vi "save_infos_v4_svi.vi"(0 "Refnum VISA en entrée":refnum<visa-resource-name>, 1 "STAGE_SPEED":dbl, 2 "info Directory":path, 3 "USED_FILTERS":u8[](array[numeric]), 4 "NUM_POS":u32, 5 "NB_CHANELS":u32, 6 "NSCAN":u32, 7 "Noff_fluidix":u32, 8 "Camera infos":string, 9 "BETWEEN_SCAN":u32, 10 "ROMODE":u32, 11 "Non_fluidix":u32, 12 "BIN":u16, 13 "useLASER":bool, 14 "SOFT_VERSION":string, 15 "Nstart_fluidics":u32, 16 "EXPT":dbl, 17 "MIN SCAN DURATION":dbl, 18 "USED_LEDS":bool[][](array[boolean]), 19 "useFLUIDCS":bool, 20 "Noff_laser":u32, 21 "Non_laser":u32, 22 "Nstart_laser":u32, 23 "BETWEEN_PATTERN":u32, 24 "NPATTERN":u32, 25 "SHOOT_AT_SCAN":u32, 26 "SHOOT_DUR":dbl, 27 "is_singleshoot":bool) -> ()   [LabVIEW 2013]
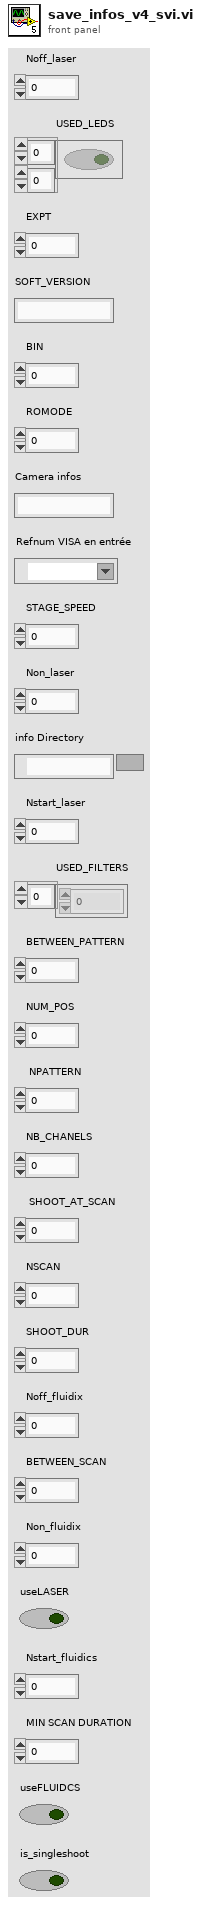
[diagram p1: front panel]
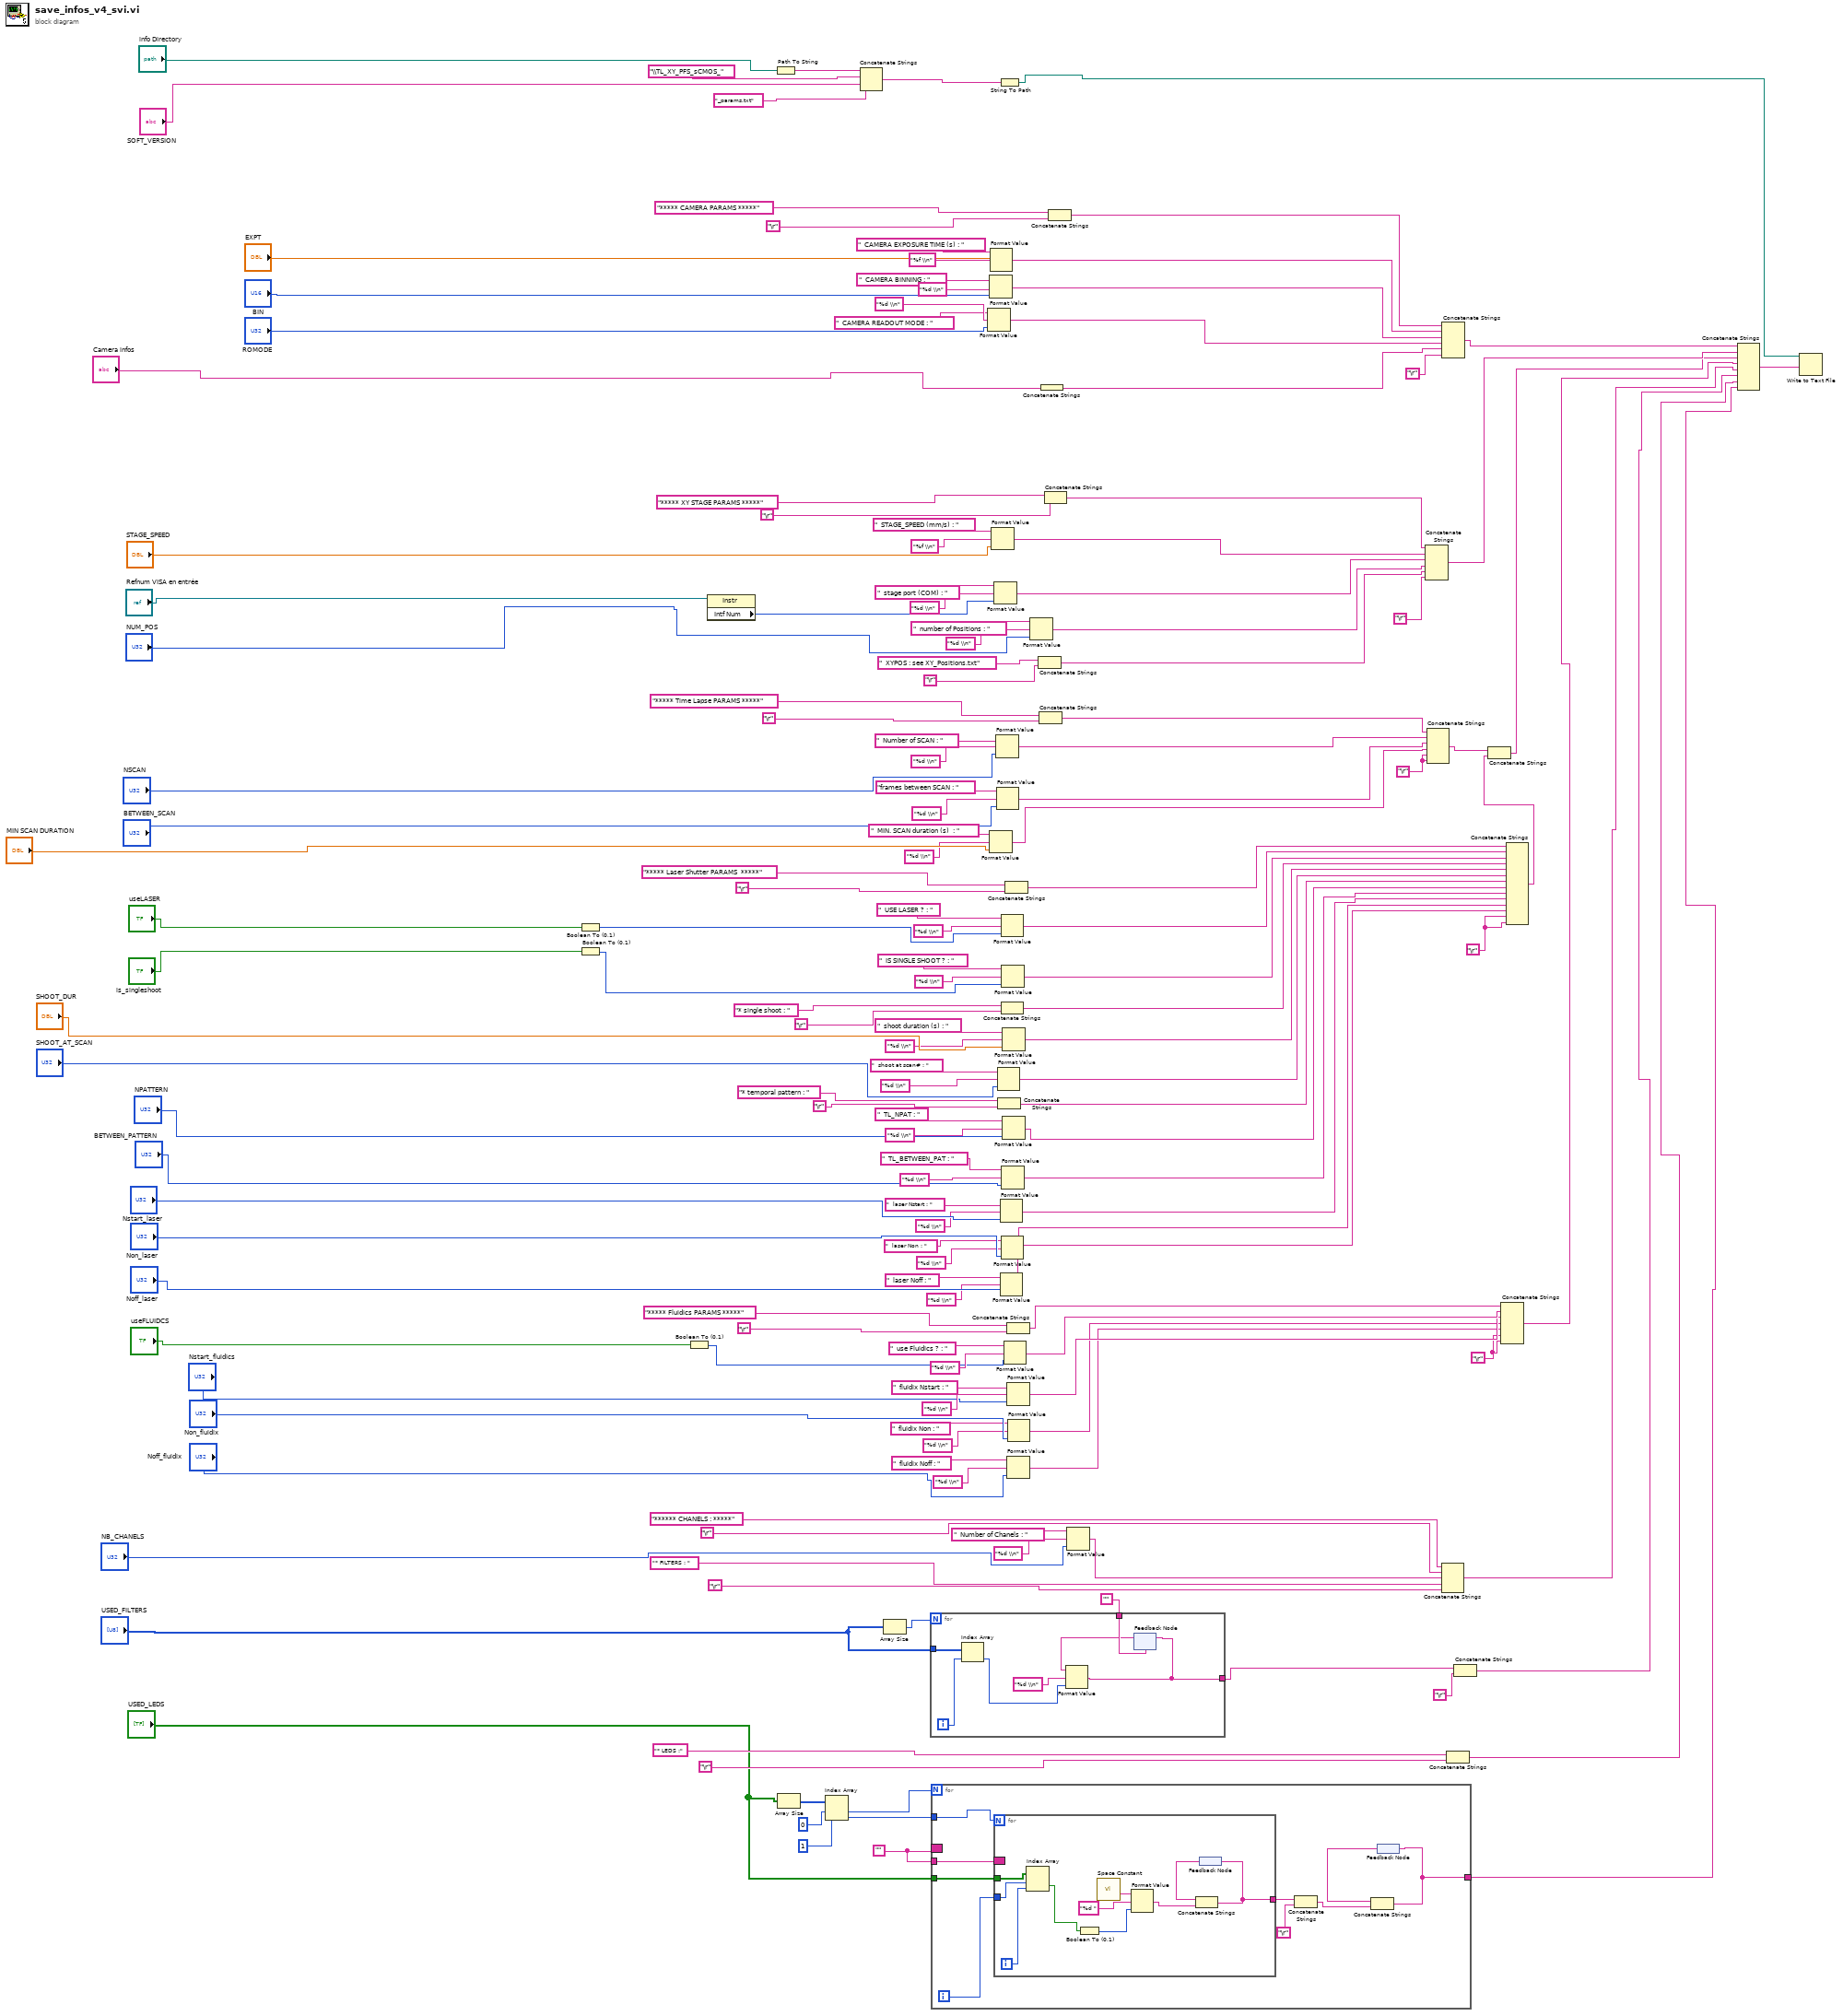
[diagram p0: block diagram]
diagram:
  w159 = "\r"
  w17 = "\r"
  w16 = "\r"
  w148 = ""
  n1 = Boolean To (0,1)(Boolean="useLASER") -> (0, 1=w56:i16)
  n2 = Boolean To (0,1)(Boolean="is_singleshoot") -> (0, 1=w55:i16)
  n3 = Boolean To (0,1)(Boolean="useFLUIDCS") -> (0, 1=w41:i16)
  n4 = property class="Instr"(reference="Refnum VISA en entrée") -> ("Intf Num"=w87:u16)  [unwired: 1 in, 2 out]
  n5 = Path To String(path="info Directory") -> (string=w70:string)
  n6 = Array Size(array="USED_LEDS") -> (size(s)=w125:i32[])
  n7 = Index Array(array=w125, index #1=0, index #2=1) -> (element #1=w126:i32, element #2=w147:i32)
  n8 = Concatenate Strings(w70, "\\TL_XY_PFS_sCMOS_", "SOFT_VERSION", "_params.txt") -> (w74:string)
  n9 = Array Size(array="USED_FILTERS") -> (size(s)=w120:i32)
  n10 = for {
    N: w120 -> [_]
    tunnel: "USED_FILTERS" -> [w168]
    tunnel: "" -> [w166]
    tunnel: [w164] -> w14
    i -> [w169]
    n11 = Index Array(array=w168, index=w169) -> (element=w167:u8)
    n12 = feedback #1(w166) -> (w165:string)
    n13 = Format Value(string ("")=w165, format string="%d \\n", value (0)=w167) -> (output string=w164:string)
    n14 = feedback-in #1(w164) -> ()
  }
  n15 = for {
    N: w126 -> [_]
    tunnel: "USED_LEDS" -> [w179]
    tunnel: [w173] -> w21
    tunnel: w147 -> [w172]
    border: w148 -> [_]
    tunnel: w148 -> [w171]
    i -> [w178]
    n16 = for {
      N: w172 -> [_]
      tunnel: w179 -> [w188]
      tunnel: w178 -> [w180]
      tunnel: [w182] -> w176
      border: w171 -> [_]
      i -> [w181]
      n17 = Index Array(array=w188, index (row)=w180, index (col)=w181) -> (element=w186:bool)
      n18 = Boolean To (0,1)(Boolean=w186) -> (0, 1=w185:i16)
      n19 = call <vilib>:"Space Constant.vi"() -> ("String"=w187:string)
      n20 = Format Value(string ("")=w187, format string="%d ", value (0)=w185) -> (output string=w184:string)
      n21 = feedback #2() -> (w183:string)
      n22 = Concatenate Strings(w183, w184) -> (w182:string)
      n23 = feedback-in #2(w182) -> ()
    }
    n24 = Concatenate Strings(w176, "\r") -> (w175:string)
    n25 = feedback #3() -> (w174:string)
    n26 = Concatenate Strings(w174, w175) -> (w173:string)
    n27 = feedback-in #3(w173) -> ()
  }
  n28 = Format Value(string ("")="  CAMERA READOUT MODE : ", format string="%d \\n", value (0)="ROMODE") -> (output string=w139:string)
  n29 = Format Value(string ("")="  CAMERA BINNING : ", format string="%d \\n", value (0)="BIN") -> (output string=w138:string)
  n30 = Format Value(string ("")="  MIN. SCAN duration (s)  : ", format string="%d \\n", value (0)="MIN SCAN DURATION") -> (output string=w160:string)
  n31 = Format Value(string ("")="  CAMERA EXPOSURE TIME (s) : ", format string="%f \\n", value (0)="EXPT") -> (output string=w137:string)
  n32 = Format Value(string ("")="  STAGE_SPEED (mm/s) : ", format string="%f \\n", value (0)="STAGE_SPEED") -> (output string=w135:string)
  n33 = Format Value(string ("")="  stage port (COM) : ", format string="%d \\n", value (0)=w87) -> (output string=w27:string)
  n34 = Format Value(string ("")="  Number of SCAN : ", format string="%d \\n", value (0)="NSCAN") -> (output string=w66:string)
  n35 = Format Value(string ("")="frames between SCAN : ", format string="%d \\n", value (0)="BETWEEN_SCAN") -> (output string=w65:string)
  n36 = Format Value(string ("")="  shoot at scan# : ", format string="%d \\n", value (0)="SHOOT_AT_SCAN") -> (output string=w38:string)
  n37 = Concatenate Strings("* temporal pattern : ", "\r") -> (w39:string)
  n38 = String To Path(string=w74) -> (path=w143:path)
  n39 = Format Value(string ("")="  laser Nstart : ", format string="%d \\n", value (0)="Nstart_laser") -> (output string=w131:string)
  n40 = Format Value(string ("")="  laser Noff : ", format string="%d \\n", value (0)="Noff_laser") -> (output string=w133:string)
  n41 = Format Value(string ("")="  USE LASER ? : ", format string="%d \\n", value (0)=w56) -> (output string=w34:string)
  n42 = Concatenate Strings("* single shoot : ", "\r") -> (w36:string)
  n43 = Format Value(string ("")="  laser Non : ", format string="%d \\n", value (0)="Non_laser") -> (output string=w132:string)
  n44 = Format Value(string ("")="  IS SINGLE SHOOT ? : ", format string="%d \\n", value (0)=w55) -> (output string=w35:string)
  n45 = Format Value(string ("")="  TL_BETWEEN_PAT : ", format string="%d \\n", value (0)="BETWEEN_PATTERN") -> (output string=w130:string)
  n46 = Format Value(string ("")="  shoot duration (s) : ", format string="%d \\n", value (0)="SHOOT_DUR") -> (output string=w37:string)
  n47 = Format Value(string ("")="  TL_NPAT : ", format string="%d \\n", value (0)="NPATTERN") -> (output string=w129:string)
  n48 = Format Value(string ("")="  use Fluidics ? : ", format string="%d \\n", value (0)=w41) -> (output string=w31:string)
  n49 = Concatenate Strings("***** Laser Shutter PARAMS  *****", "\r") -> (w33:string)
  n50 = Concatenate Strings("***** Fluidics PARAMS *****", "\r") -> (w32:string)
  n51 = Format Value(string ("")="  fluidix Nstart : ", format string="%d \\n", value (0)="Nstart_fluidics") -> (output string=w30:string)
  n52 = Format Value(string ("")="  fluidix Noff : ", format string="%d \\n", value (0)="Noff_fluidix") -> (output string=w28:string)
  n53 = Format Value(string ("")="  fluidix Non : ", format string="%d \\n", value (0)="Non_fluidix") -> (output string=w29:string)
  n54 = Format Value(string ("")="  number of Positions : ", format string="%d \\n", value (0)="NUM_POS") -> (output string=w9:string)
  n55 = Concatenate Strings("  XYPOS : see XY_Positions.txt", "\r") -> (w8:string)
  n56 = Concatenate Strings("***** Time Lapse PARAMS *****", "\r") -> (w67:string)
  n57 = Concatenate Strings("Camera infos") -> (w26:string)
  n58 = Concatenate Strings("***** XY STAGE PARAMS *****", "\r") -> (w134:string)
  n59 = Concatenate Strings("***** CAMERA PARAMS *****", "\r") -> (w136:string)
  n60 = Format Value(string ("")="  Number of Chanels : ", format string="%d \\n", value (0)="NB_CHANELS") -> (output string=w1:string)
  n61 = Concatenate Strings(w134, w135, w27, w9, w8, "\r") -> (w141:string)
  n62 = Concatenate Strings(w67, w66, w65, w160, w159, w159) -> (w20:string)
  n63 = Concatenate Strings("****** CHANELS : *****", "\r", w1, "* FILTERS : ", "\r") -> (w23:string)
  n64 = Concatenate Strings(w136, w137, w138, w139, w26, "\r") -> (w140:string)
  n65 = Concatenate Strings("* LEDS :", "\r") -> (w22:string)
  n66 = Concatenate Strings(w14, "\r") -> (w13:string)
  n67 = Concatenate Strings(w32, w31, w30, w29, w28, w16, w16) -> (w24:string)
  n68 = Concatenate Strings(w33, w34, w35, w36, w37, w38, w39, w129, w130, w131, w132, w133, w17, w17) -> (w19:string)
  n69 = Concatenate Strings(w20, w19) -> (w18:string)
  n70 = Concatenate Strings(w140, w141, w18, w24, w23, w13, w22, w21) -> (w142:string)
  n71 = Write to Text File(file (use dialog)=w143, text=w142) -> ()  [unwired: 2 in, 3 out]
